vi "Motion.vi"() -> ()   [LabVIEW 2022 SP3]
uses:
  <vilib>/DAQmx/read.llb/DAQmx Read (Analog DBL 1Chan 1Samp).vi
  <vilib>/DAQmx/write.llb/DAQmx Write (Digital Bool 1Line 1Point).vi
  <vilib>/DAQmx/create/channels.llb/DAQmx Create Channel (AI-Voltage-Basic).vi
  <vilib>/DAQmx/create/channels.llb/DAQmx Create Channel (DO-Digital Output).vi
  <vilib>/DAQmx/miscellaneous.llb/DAQmx Fill In Error Info.vi
panel:
  out "Waveform Chart":dbl(graph)
  out "Numeric":dbl
  in  "lines":tag
  in  "stop 2":bool
  out "Voltage":dbl(knob) scale=0.0..10.0
  in  "stop":bool
  in  "physical channels":tag
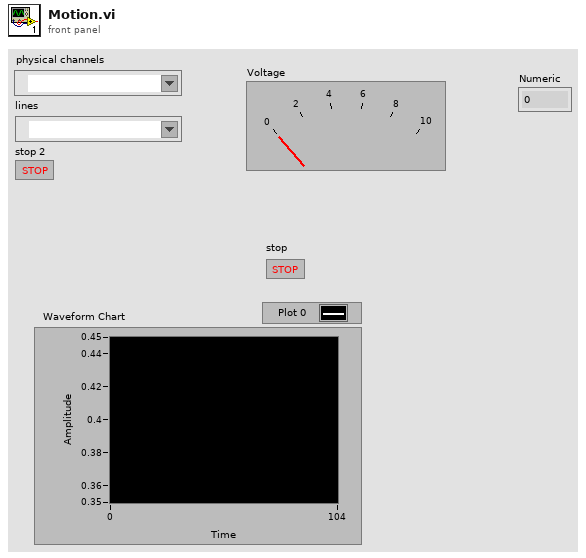
[diagram p1: front panel]
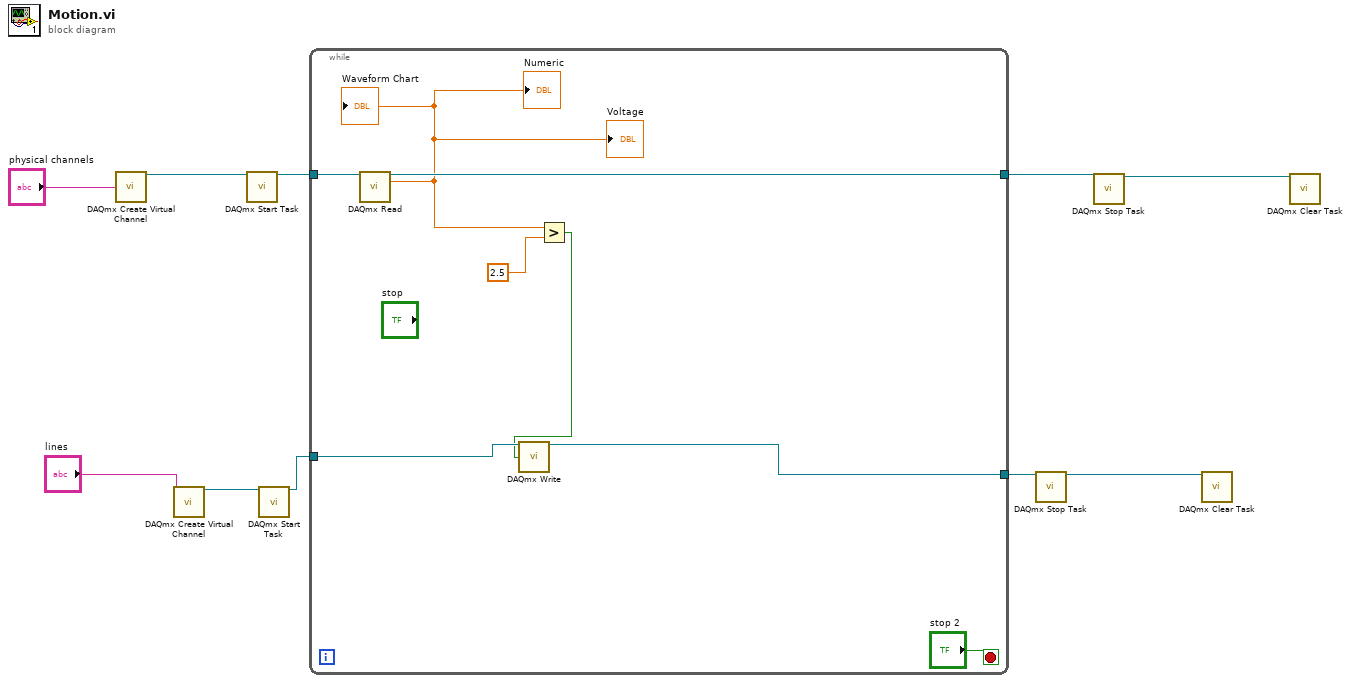
[diagram p0: block diagram]
diagram:
  n1 = call-poly <vilib>:"DAQmx Create Virtual Channel.vi"("physical channels"="physical channels") -> ("task out"=w9:refnum<k21>)  [unwired: 13 in, 1 out]
  n2 = call-poly <vilib>:"DAQmx Create Virtual Channel.vi"("lines"="lines") -> ("task out"=w2:refnum<k21>)  [unwired: 13 in, 1 out]
  n3 = call <vilib>:"DAQmx Start Task.vi"("task/channels in"=w9) -> ("task out"=w8:refnum<k21>)  [unwired: 13 in, 1 out]
  n4 = call <vilib>:"DAQmx Start Task.vi"("task/channels in"=w2) -> ("task out"=w5:refnum<k21>)  [unwired: 13 in, 1 out]
  n5 = while {
    tunnel: w8 -> [w18]
    tunnel: [w17] -> w6
    tunnel: w5 -> [w15]
    tunnel: [w14] -> w4
    stop <- "stop 2" stop-if-true
    n6 = call-poly <vilib>:"DAQmx Read.vi"("task/channels in"=w18) -> ("task out"=w17:refnum<k21>, "data"=w11:dbl)  [unwired: 12 in, 1 out]
    "Voltage" <- w11
    "Numeric" <- w11
    "Waveform Chart" <- w11
    n7 = Greater?(x=w11, y=2.5) -> (0:w12:bool)
    n8 = call-poly <vilib>:"DAQmx Write.vi"("task/channels in"=w15, "data"=w12) -> ("task out"=w14:refnum<k21>)  [unwired: 11 in, 2 out]
  }
  n9 = call <vilib>:"DAQmx Stop Task.vi"("task/channels in"=w4) -> ("task out"=w3:refnum<k21>)  [unwired: 13 in, 1 out]
  n10 = call <vilib>:"DAQmx Stop Task.vi"("task/channels in"=w6) -> ("task out"=w7:refnum<k21>)  [unwired: 13 in, 1 out]
  n11 = call <vilib>:"DAQmx Clear Task.vi"("task in"=w3) -> ()  [unwired: 14 in, 1 out]
  n12 = call <vilib>:"DAQmx Clear Task.vi"("task in"=w7) -> ()  [unwired: 14 in, 1 out]
